vi "PlotRovers.vi"(3 "Fill Color":u32(colorbox)=16734710, 4 "Position Array":i32[][](array[numeric])=[[200, 200], [200, 800], [800, 800], [800, 200], [500, 300], [895, 748], [330, 598], [300, 200], [350, 200]], 5 "Picture In":picture) -> (2 "Picture Out":picture)   [LabVIEW 2012]
panel:
  in  "Heading":dbl
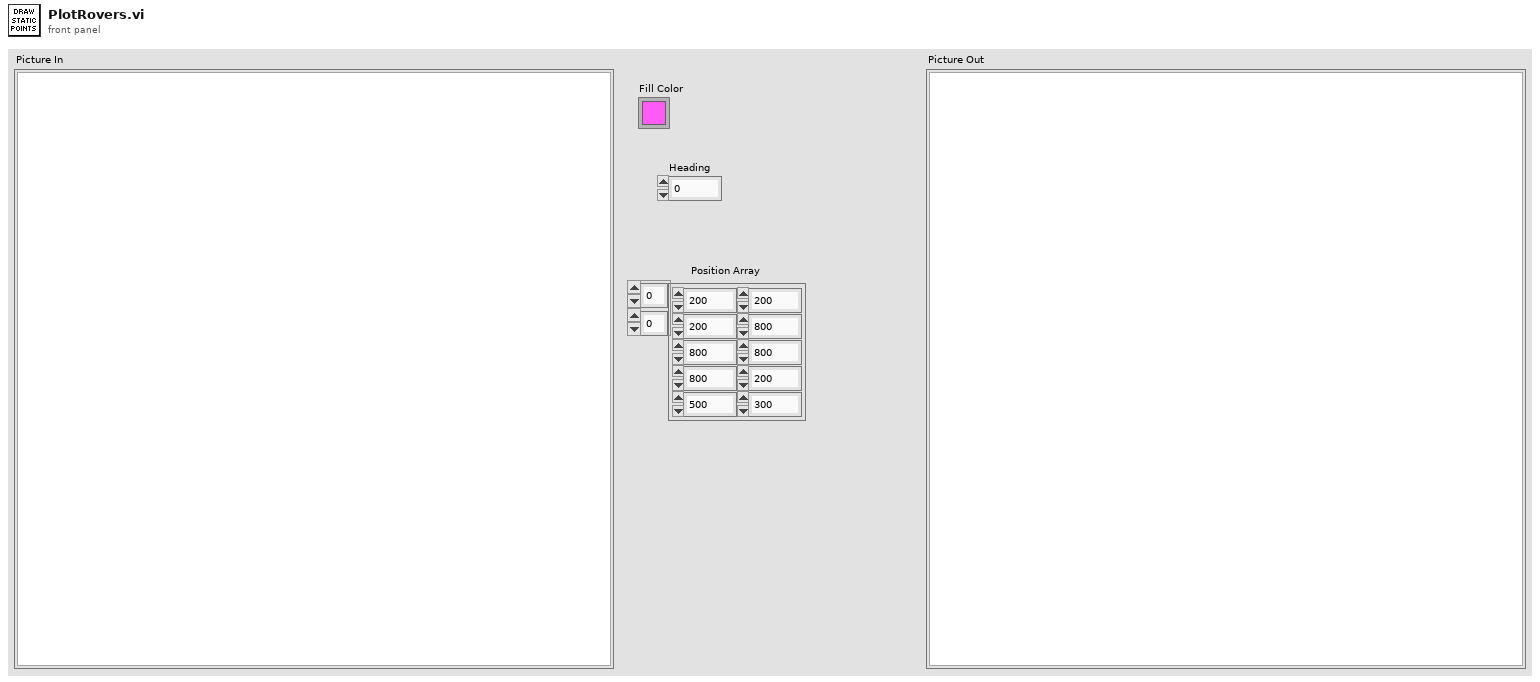
[diagram p1: front panel]
types:
  T1 = cluster{"[0]":i16, "[1]":i16, "[2]":i16, "[3]":i16, "[4]":i16, "[5]":i16, "[6]":i16, "[7]":i16, "[8]":i16}
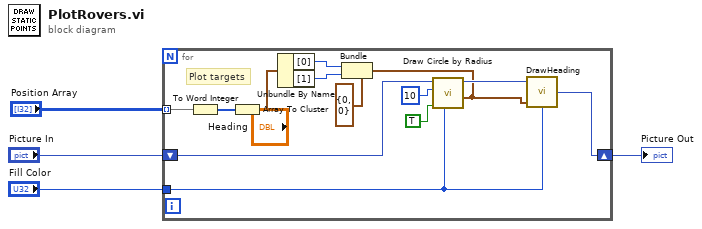
[diagram p0: block diagram]
diagram:
  n1 = for {
    shift-right: [w6] -> w3
    shift-left: "Picture In" -> [w9]
    tunnel: "Position Array" -> [w15] mode=indexing
    tunnel: "Fill Color" -> [w5]
    # "Plot targets"
    n2 = To Word Integer(number=w15) -> (16bit integer=w14:i16[])
    n3 = Array To Cluster(array=w14) -> (cluster=w13:T1)
    n4 = Unbundle By Name(w13) -> ("[0]"=w12:i16, "[1]"=w11:i16)
    n5 = Bundle(cluster=cluster{i16, i16} {0, 0} ("input cluster"), w12, w11) -> (w7:cluster{i16, i16})
    n6 = call <vilib>:"Draw Circle by Radius.vi"("color(black)"=w5, "fill?(F)"=TRUE, "pixel center"=w7, "radius"=i16 10, "picture"=w9) -> ("new picture"=w8:picture)  [unwired: 6 in]
    n7 = call "DrawHeading.vi"("color(black)"=w5, "(xr,yr) old"=w7, "2D Picture"=w8) -> ("new picture"=w6:picture)  [unwired: 1 in]
  }
  "Picture Out" <- w3
